vi "display_michelle_PKT_visjitter_stopadded_RandCont_PsuedoCO_TSLogFC2_ForTrainingLT.vi"() -> ()   [LabVIEW 2019]
uses:
  <vilib>/Analysis/Matrix/Datatypes/RealMatrix.ctl
  <vilib>/Utility/miscctls.llb/LVDateTimeRec.ctl
  <vilib>/Utility/file.llb/Write Delimited Spreadsheet (DBL).vi
  <vilib>/Analysis/Matrix/NI_Matrix.lvlib
panel:
  out "TimeStampTime":dbl
  out "initiatedlag":dbl
  out "date time rec":T1
  out "GlobalStartTime":i32
  out "JustStarted":i32
  out "LastTimeOutTime":dbl
  out "lambda":dbl
  out "maxITI":dbl
  out "minITI":dbl
  out "goEXP":dbl
  out "meanITI":dbl
  out "Lag1":dbl
  out "TSLog":dbl[][](array[numeric])
  out "TSLog2":dbl[][](array[numeric])
  out "Initialtime":dbl
  out "TSLog1":dbl[][](array[numeric])
  out "ArrayTemp3":T2
  out "StimID2":dbl
  out "Contrast":dbl
  out "TimeOutCounter":i32
  out "ElapsedTime_M":dbl
  out "Base_Contrast":dbl
  out "CurrentTrial":u32=1
  out "Jitter":dbl
  out "BaseITI":dbl
  out "VisStimDuration":dbl
  in  "Stop":bool
  out "Num trials":u32=204
  out "ISI Time":dbl
  out "Stim TS":dbl
  out "Output":dbl[][](array[numeric])
  out "Output frame":T2
  out "Array temp1":T2
  out "Elapsed Time":dbl
  out "Display":bool=TRUE
  out "Trial":u32=1
  out "reward":dbl[](array[numeric])
  out "stim_id":dbl[](array[numeric])
  out "stim_loaded":dbl
  out "Timings":dbl[](array[numeric])
  out "Stimuli Loaded?":bool
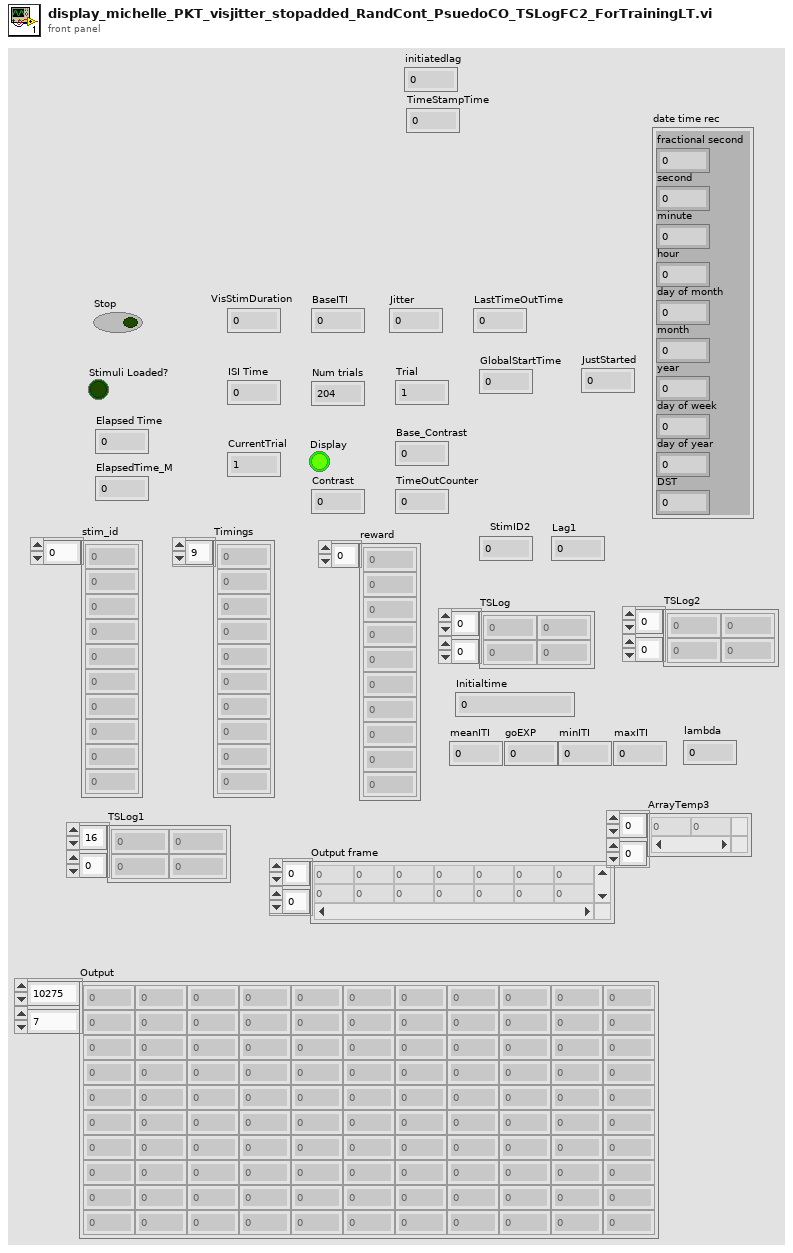
[diagram p1: front panel]
types:
  T1 = typedef "LVDateTimeRec.ctl" = cluster{"fractional second":dbl, "second":i32, "minute":i32, "hour":i32, "day of month":i32, "month":i32, "year":i32, "day of week":i32, "day of year":i32, "DST":i32}
  T2 = typedef "NI_Matrix.lvlib/RealMatrix.ctl" = dbl[][]
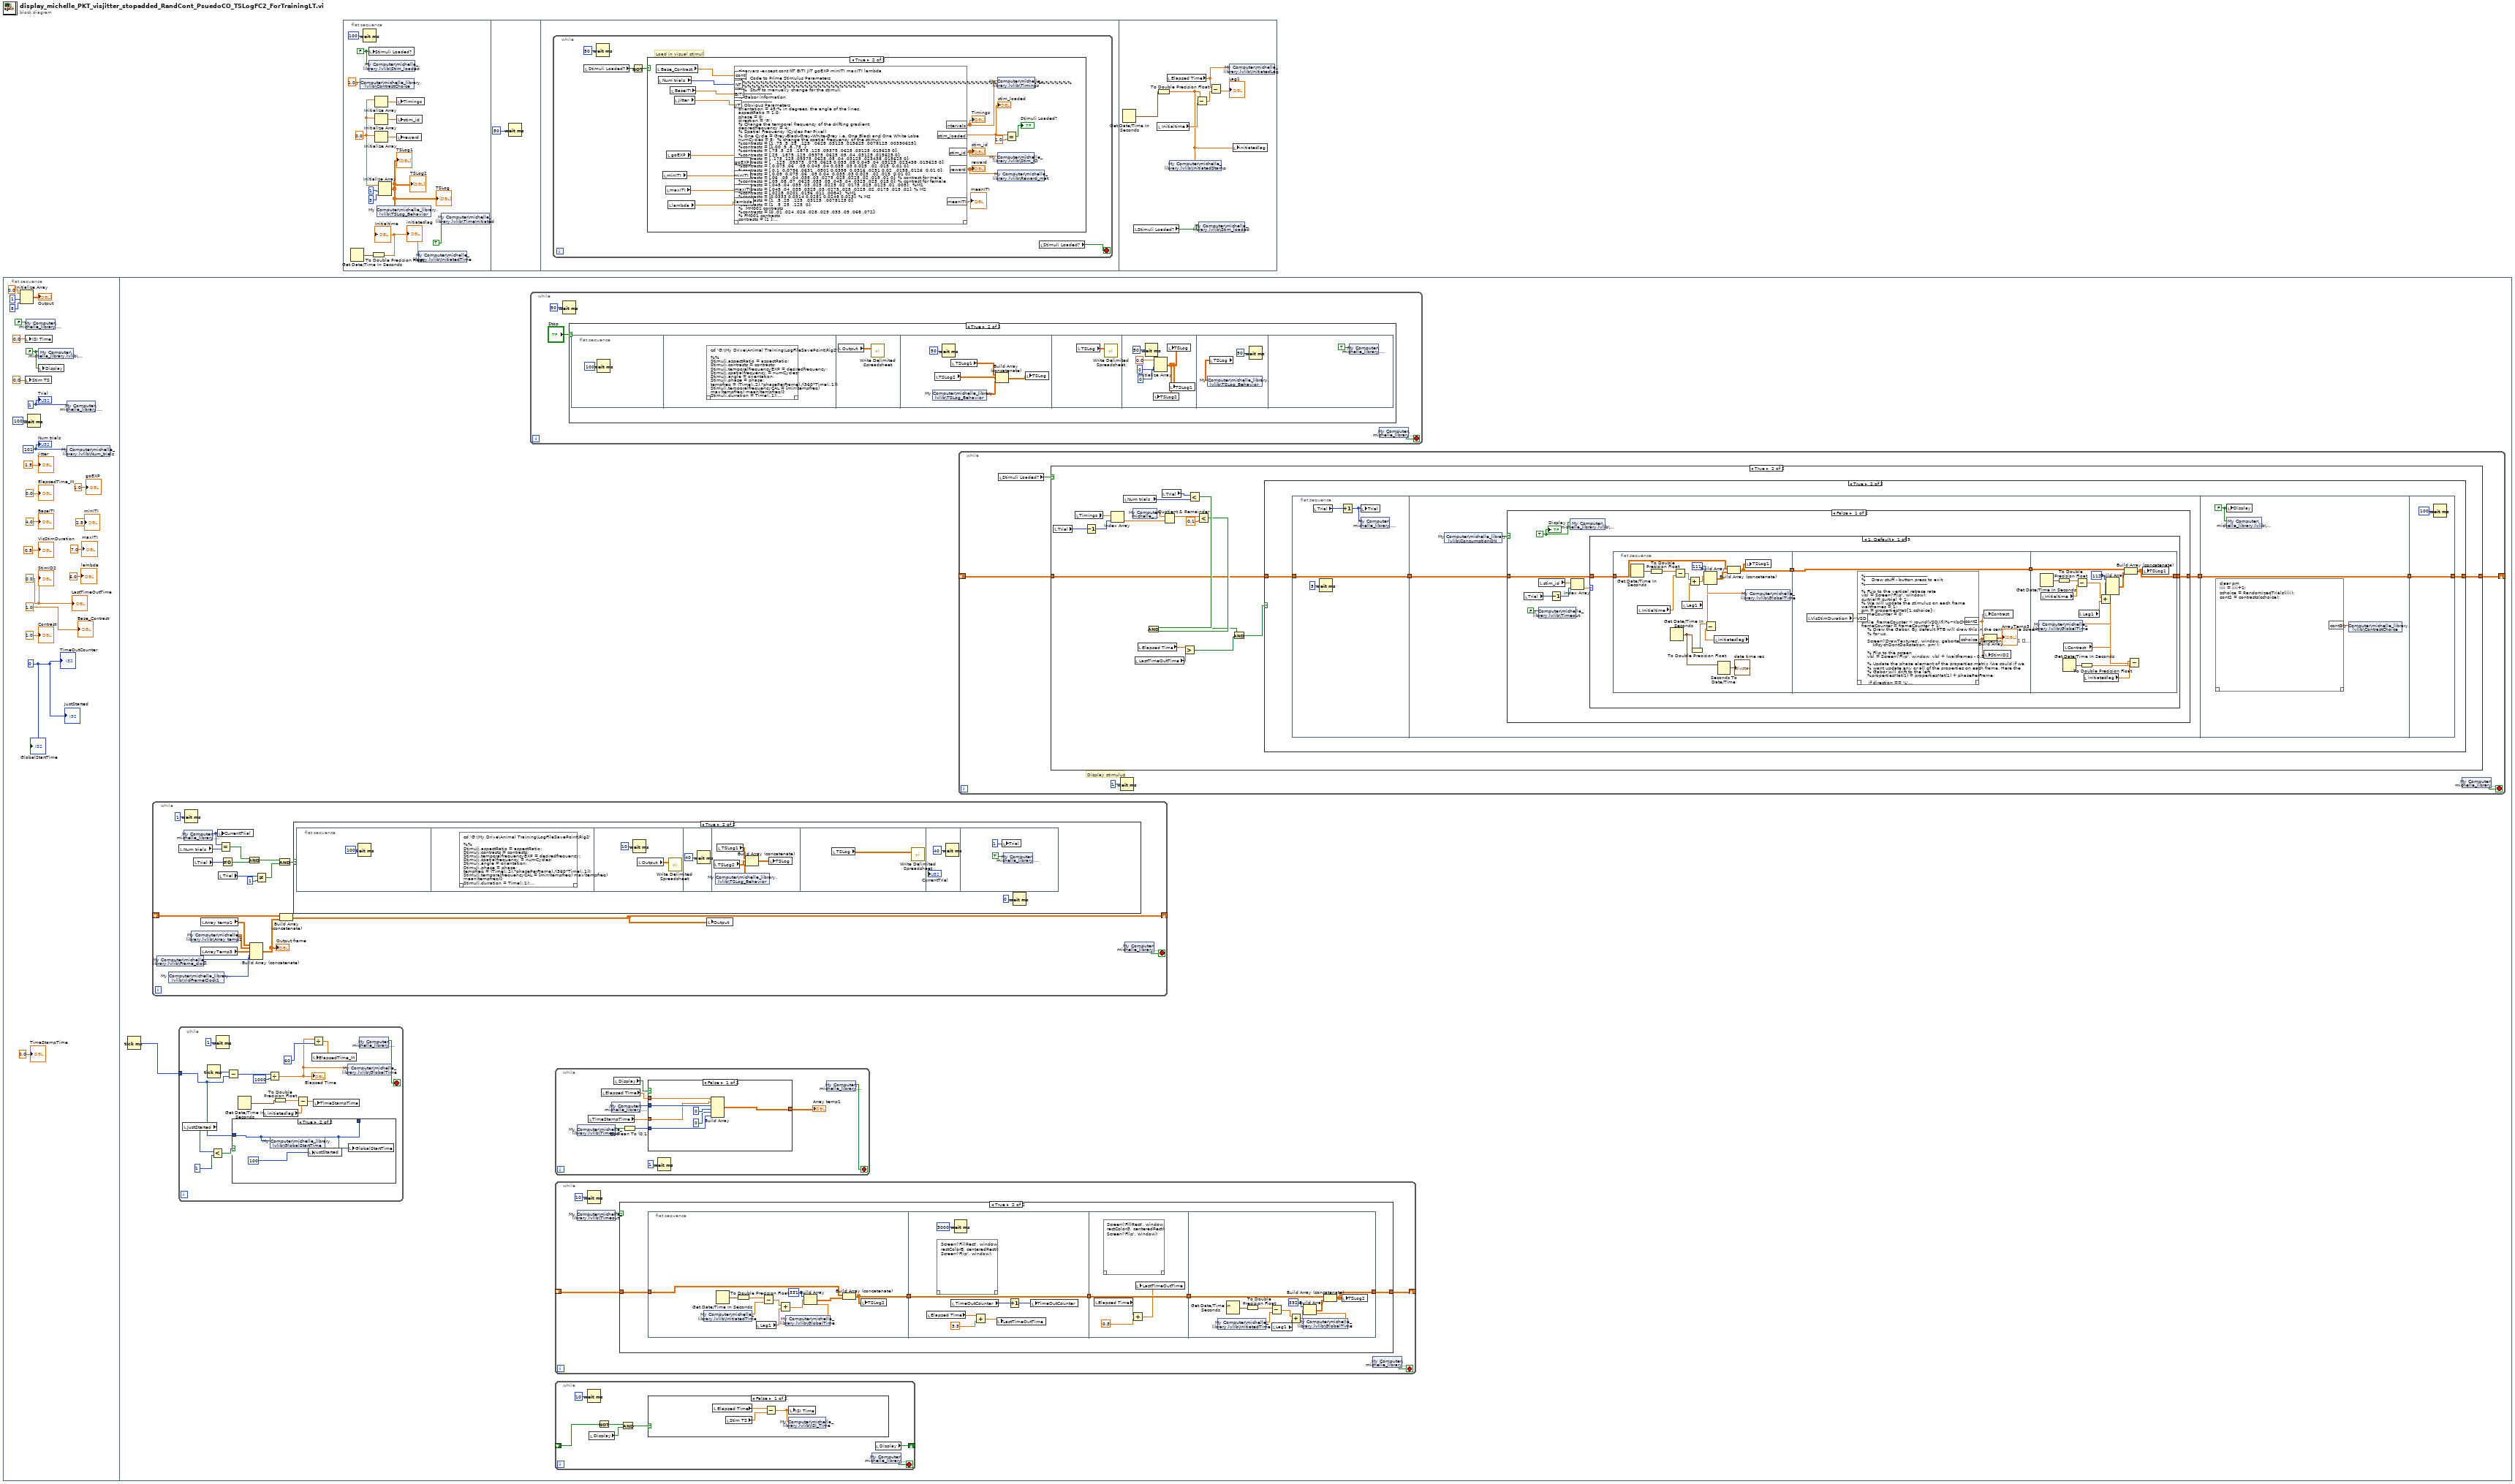
[diagram p0: block diagram]
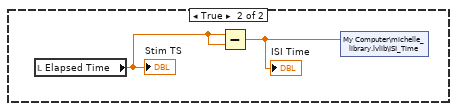
[diagram p5: hidden frame]
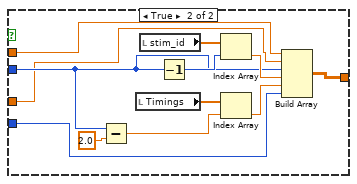
[diagram p6: hidden frame]
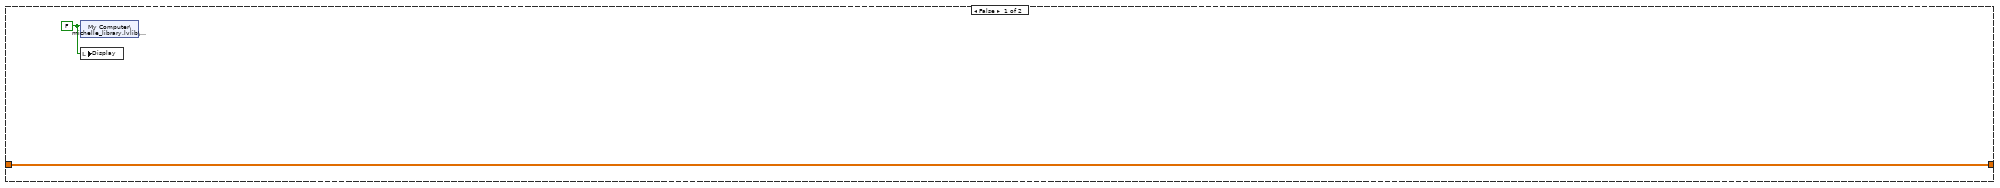
[diagram p10: hidden frame]
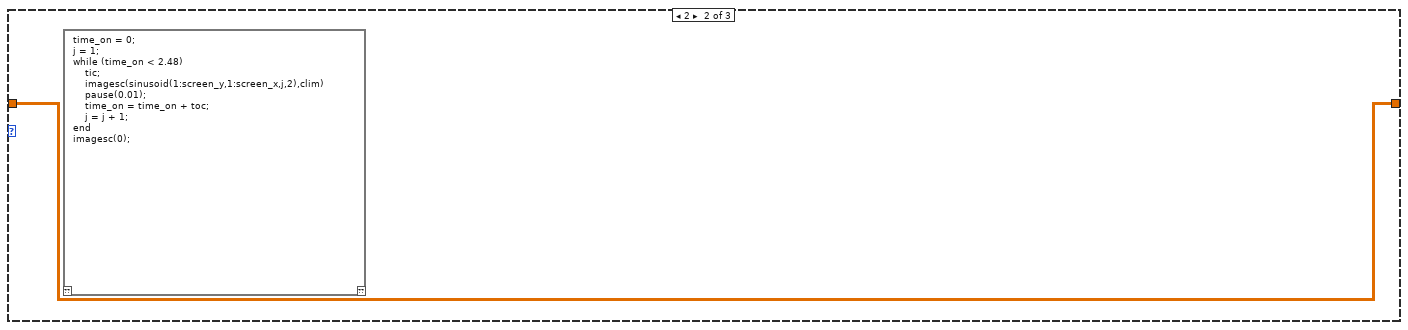
[diagram p11: hidden frame]
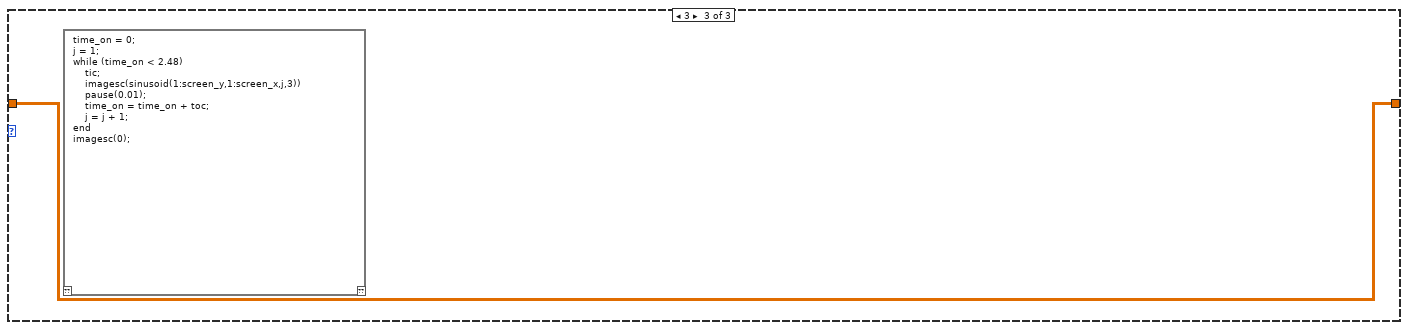
[diagram p12: hidden frame]
diagram:
  n1 = flat-sequence {
    frame #0 {
      w2 = 0.0
      w8 = 0
      w16 = u32 101
      w22 = FALSE ("Display")
      w24 = u32 1 ("Trial")
      n2 = Initialize Array(0.0 ("element"), 1 ("dimension size"), 8 ("dimension size")) -> (→"Output":dbl[][])
      n3 = local write "ISI Time"(0.0 ("ISI Time")) -> ()
      n4 = local write "Stim TS"(0.0 ("Stim TS")) -> ()
      n5 = shared-variable "My Computer\\michelle_library.lvlib\\Stop"(FALSE ("Stop")) -> ()  [unwired: 1 in, 1 out]
      n6 = Wait (ms)(milliseconds to wait=u32 100) -> ()  [unwired: 1 out]
      n7 = shared-variable "My Computer\\michelle_library.lvlib\\Display"(w22) -> ()  [unwired: 1 in, 1 out]
      n8 = local write "Display"(w22) -> ()
      n9 = shared-variable "My Computer\\michelle_library.lvlib\\Trial"(w24) -> ()  [unwired: 1 in, 1 out]
      n10 = shared-variable "My Computer\\michelle_library.lvlib\\Num_trials"(w16) -> ()  [unwired: 1 in, 1 out]
      "Trial" <- w24
      "Num trials" <- w16
      "VisStimDuration" <- 0.5
      "BaseITI" <- 4.0
      "Jitter" <- 1.5
      "Base_Contrast" <- 1.0
      "ElapsedTime_M" <- 0.0
      "TimeOutCounter" <- w8
      "Contrast" <- 1.0
      "StimID2" <- w2
      "goEXP" <- 1.0
      "minITI" <- 2.5
      "maxITI" <- 7.0
      "lambda" <- 6.0
      "LastTimeOutTime" <- w2
      "JustStarted" <- w8
      "GlobalStartTime" <- w8
      "TimeStampTime" <- 0.0
    }
    frame #1 {
      n11 = Tick Count (ms)() -> (millisecond timer value=w25:u32)
      n12 = while {
        shift-right: [w164] -> _
        shift-left: _ -> [w165]
        stop <- w167 stop-if-true
        n13 = shared-variable "My Computer\\michelle_library.lvlib\\Frame_clock"() -> (w149:u32)  [unwired: 1 in, 1 out]
        n14 = shared-variable "My Computer\\michelle_library.lvlib\\VidFrameClock1"() -> (w148:u32)  [unwired: 1 in, 1 out]
        n15 = local read "Num trials"() -> (w160:u32)
        n16 = shared-variable "My Computer\\michelle_library.lvlib\\Trial"() -> (w151:u32)  [unwired: 1 in, 1 out]
        n17 = Wait (ms)(milliseconds to wait=u32 1) -> ()  [unwired: 1 out]
        n18 = shared-variable "My Computer\\michelle_library.lvlib\\Array temp2"() -> (w162:dbl[][])  [unwired: 1 in, 1 out]
        n19 = local read "Trial"() -> (w158:u32)
        n20 = local read "Array temp1"() -> (w163:T2)
        n21 = local read "ArrayTemp3"() -> (w150:T2)
        n22 = local write "CurrentTrial"(w151) -> ()
        n23 = local read "Trial"() -> (w157:u32)
        n24 = Equal?(x=w151, y=w160) -> (x = y?=w159:bool)
        n25 = Not Equal To 0?(x=w158) -> (x != 0?=w154:bool)
        n26 = And(x=w159, y=w154) -> (x .and. y?=w152:bool)
        n27 = Build Array (concatenate)(w163, w162, w150, w149, w148) -> (w161:T2)
        "Output frame" <- w161
        n28 = Not Equal?(x=w157, y=1) -> (x != y?=w156:bool)
        n29 = And(x=w152, y=w156) -> (x .and. y?=w153:bool)
        n30 = Build Array (concatenate) ("Build Matrix")(w165, w161) -> (w164:T2)
        n31 = case shown="True" w153 {
          frame False {
          }
          frame True {
            n32 = flat-sequence {
              frame #0 {
                n33 = Wait (ms)(milliseconds to wait=100) -> ()  [unwired: 1 out]
              }
              frame #1 {
                n34 = script code="cd 'G:\\My Drive\\Animal Training\\LogFileSavePoint\\Rig2'\n\n%%\nStimuli.aspectRatio = aspectRatio;\nStimuli.contrasts = contrasts;\nStimuli.temporalfrequencyEXP = desiredfrequency;\nStimuli.spatialfrequency = numCycles;\nStimuli.angle = orientation;\nStimuli.phase = phase;\ntempfreq = (Time(:,2).*phasePerFrame)./(360*Time(:,1)); \nStimuli.temporalfrequencyCAL = [min(tempfreq) max(tempfreq) mean(tempfreq)];\nStimuli.durration = Time(:,1);\nStimuli.frames = Time(:,2);\nStimuli.contrast = Time(:,3);\nStimuli.intervals = intervals;\nif goEXP == 0\n     int.type = 'jitter';\n     int.baseITI = BITI;\n     int.jitter = JIT;\nelseif goEXP == 1\n     int.type = 'exponential';\n     int.minITI = minITI;\n     int.maxITI = maxITI;\n     int.lambda = lambda;\nend\nStimuli.IntervalData = int;\n\n\nWindow.Xpixels = screenXpixels;\nWindow.Ypixels = screenYpixels;\nWindow.Xcenter = xCenter;\nWindow.Ycenter = yCenter;\nWindow.ifi = ifi;\nWindow.screen = screenNumber;\n\n%%\n[logname] = generatelogname();\n\nsave(logname,'Stimuli','Window');"() -> ()  [unwired: 1 in, 1 out]
              }
              frame #2 {
                n35 = Wait (ms)(milliseconds to wait=u32 10) -> ()  [unwired: 1 out]
                n36 = local read "Output"() -> (w171:dbl[][])
                n37 = call-poly <vilib>:"Write Delimited Spreadsheet.vi"("2D data"=w171) -> ()  [unwired: 13 in, 2 out]
              }
              frame #3 {
                n38 = Wait (ms)(milliseconds to wait=u32 40) -> ()  [unwired: 1 out]
              }
              frame #4 {
                n39 = local read "TSLog2"() -> (w176:dbl[][])
                n40 = shared-variable "My Computer\\michelle_library.lvlib\\TSLog_Behavior"() -> (w174:dbl[][])  [unwired: 1 in, 1 out]
                n41 = local read "TSLog1"() -> (w175:dbl[][])
                n42 = Build Array (concatenate) ("Build Matrix")(w175, w176, w174) -> (w173:T2)
                n43 = local write "TSLog"(w173) -> ()
              }
              frame #5 {
                n44 = local read "TSLog"() -> (w177:dbl[][])
                n45 = call-poly <vilib>:"Write Delimited Spreadsheet.vi"("2D data"=w177) -> ()  [unwired: 13 in, 2 out]
              }
              frame #6 {
                n46 = Wait (ms)(milliseconds to wait=u32 40) -> ()  [unwired: 1 out]
              }
              frame #7 {
                n47 = local write "Trial"(1) -> ()
                n48 = shared-variable "My Computer\\michelle_library.lvlib\\Stop"(TRUE) -> ()  [unwired: 1 in, 1 out]
              }
            }
            n49 = Wait (ms)(milliseconds to wait=0) -> ()  [unwired: 1 out]
          }
        }
        n50 = local write "Output"(w164) -> ()
        n51 = shared-variable "My Computer\\michelle_library.lvlib\\Stop"() -> (w167:bool)  [unwired: 1 in, 1 out]
      }
      n52 = while {
        tunnel: w25 -> [w133]
        stop <- w140 stop-if-true
        n53 = local read "JustStarted"() -> (w135:i32)
        n54 = Tick Count (ms)() -> (millisecond timer value=w143:u32)
        n55 = Less?(x=w135, y=1) -> (x < y?=w136:bool)
        n56 = Wait (ms)(milliseconds to wait=u32 1) -> ()  [unwired: 1 out]
        n57 = Subtract(x=w143, y=w133) -> (x-y=w141:u32)
        n58 = case shown="True" w136 {
          tunnel: w133 -> [w145 w146]
          tunnel: [w145 w146] -> _
          frame False {
          }
          frame True {
            n59 = shared-variable "My Computer\\michelle_library.lvlib\\GlobalStartTime"(w146) -> ()  [unwired: 1 in, 1 out]
            n60 = local write "JustStarted"(100) -> ()
            n61 = local write "GlobalStartTime"(w146) -> ()
          }
        }
        n62 = Get Date/Time In Seconds() -> (seconds since 1Jan1904=w132:timestamp)
        n63 = local read "initiatedlag"() -> (w130:dbl)
        n64 = Divide(x=w141, y=u32 1000) -> (x/y=w137:dbl)
        "Elapsed Time" <- w137
        n65 = To Double Precision Float(number=w132) -> (double precision float=w129:dbl)
        n66 = Subtract(x=w129, y=w130) -> (x-y=w131:dbl)
        n67 = Divide(x=w137, y=60) -> (x/y=w138:dbl)
        n68 = local write "ElapsedTime_M"(w138) -> ()
        n69 = local write "TimeStampTime"(w131) -> ()
        n70 = shared-variable "My Computer\\michelle_library.lvlib\\GlobalTime"(w137) -> ()  [unwired: 1 in, 1 out]
        n71 = shared-variable "My Computer\\michelle_library.lvlib\\Stop"() -> (w140:bool)  [unwired: 1 in, 1 out]
      }
      n72 = while {
        stop <- w28 stop-if-true
        n73 = Wait (ms)(milliseconds to wait=50) -> ()  [unwired: 1 out]
        n74 = case shown="True" "Stop" {
          frame False {
          }
          frame True {
            n75 = flat-sequence {
              frame #0 {
                n76 = Wait (ms)(milliseconds to wait=100) -> ()  [unwired: 1 out]
              }
              frame #1 {
                n77 = script code="cd 'G:\\My Drive\\Animal Training\\LogFileSavePoint\\Rig2'\n\n%%\nStimuli.aspectRatio = aspectRatio;\nStimuli.contrasts = contrasts;\nStimuli.temporalfrequencyEXP = desiredfrequency;\nStimuli.spatialfrequency = numCycles;\nStimuli.angle = orientation;\nStimuli.phase = phase;\ntempfreq = (Time(:,2).*phasePerFrame)./(360*Time(:,1)); \nStimuli.temporalfrequencyCAL = [min(tempfreq) max(tempfreq) mean(tempfreq)];\nStimuli.durration = Time(:,1);\nStimuli.frames = Time(:,2);\nStimuli.contrast = Time(:,3);\nStimuli.intervals = intervals;\nif goEXP == 0\n     int.type = 'jitter';\n     int.baseITI = BITI;\n     int.jitter = JIT;\nelseif goEXP == 1\n     int.type = 'exponential';\n     int.minITI = minITI;\n     int.maxITI = maxITI;\n     int.lambda = lambda;\nend\nStimuli.IntervalData = int;\n\n\nWindow.Xpixels = screenXpixels;\nWindow.Ypixels = screenYpixels;\nWindow.Xcenter = xCenter;\nWindow.Ycenter = yCenter;\nWindow.ifi = ifi;\nWindow.screen = screenNumber;\n\n%%\n[logname] = generatelogname();\n\nsave(logname,'Stimuli','Window');"() -> ()  [unwired: 1 in, 1 out]
              }
              frame #2 {
                n78 = local read "Output"() -> (w30:dbl[][])
                n79 = call-poly <vilib>:"Write Delimited Spreadsheet.vi"("2D data"=w30) -> ()  [unwired: 13 in, 2 out]
              }
              frame #3 {
                n80 = shared-variable "My Computer\\michelle_library.lvlib\\TSLog_Behavior"() -> (w31:dbl[][])  [unwired: 1 in, 1 out]
                n81 = local read "TSLog2"() -> (w34:dbl[][])
                n82 = Wait (ms)(milliseconds to wait=50) -> ()  [unwired: 1 out]
                n83 = local read "TSLog1"() -> (w33:dbl[][])
                n84 = Build Array (concatenate) ("Build Matrix")(w33, w34, w31) -> (w32:T2)
                n85 = local write "TSLog"(w32) -> ()
              }
              frame #4 {
                n86 = local read "TSLog"() -> (w36:dbl[][])
                n87 = call-poly <vilib>:"Write Delimited Spreadsheet.vi"("2D data"=w36) -> ()  [unwired: 13 in, 2 out]
              }
              frame #5 {
                n88 = Wait (ms)(milliseconds to wait=50) -> ()  [unwired: 1 out]
                n89 = Initialize Array(0.0, 0, 0) -> (w38:dbl[][])
                n90 = local write "TSLog2"(w38) -> ()
                n91 = local write "TSLog"(w38) -> ()
                n92 = local write "TSLog1"(w38) -> ()
              }
              frame #6 {
                n93 = local read "TSLog"() -> (w43:dbl[][])
                n94 = shared-variable "My Computer\\michelle_library.lvlib\\TSLog_Behavior"(w43) -> ()  [unwired: 1 in, 1 out]
                n95 = Wait (ms)(milliseconds to wait=50) -> ()  [unwired: 1 out]
              }
              frame #7 {
                n96 = shared-variable "My Computer\\michelle_library.lvlib\\Stop"(TRUE) -> ()  [unwired: 1 in, 1 out]
              }
            }
          }
        }
        n97 = shared-variable "My Computer\\michelle_library.lvlib\\Stop"() -> (w28:bool)  [unwired: 1 in, 1 out]
      }
      n98 = while {
        stop <- w104 stop-if-true
        n99 = shared-variable "My Computer\\michelle_library.lvlib\\Timeout"() -> (w102:bool)  [unwired: 1 in, 1 out]
        n100 = local read "TimeStampTime"() -> (w101:dbl)
        n101 = local read "Elapsed Time"() -> (w108:dbl)
        n102 = shared-variable "My Computer\\michelle_library.lvlib\\Trial"() -> (w106:u32)  [unwired: 1 in, 1 out]
        n103 = local read "Display"() -> (w105:bool)
        n104 = Boolean To (0,1)(Boolean=w102) -> (0, 1=w103:i16)
        n105 = case shown="False" w105 {
          tunnel: w106 -> [w116 w120]
          tunnel: w108 -> [w110 w118]
          tunnel: [w115 w127] -> w107
          tunnel: w103 -> [w112 w122]
          tunnel: w101 -> [w111 w117]
          frame False {
            n106 = Build Array(w110, w111, w116, u32 0 ("milliseconds to wait"), 0, w112) -> (w115:T2)
          }
          frame True {
            n107 = Subtract(x=w120, y=2.0) -> (x-y=w119:dbl)
            n108 = local read "Timings"() -> (w125:dbl[])
            n109 = local read "stim_id"() -> (w128:dbl[])
            n110 = Decrement(x=w120) -> (x-1=w124:u32)
            n111 = Index Array(array=w128, index=w124) -> (element=w126:dbl)
            n112 = Index Array(array=w125, index=w119) -> (element=w123:dbl)
            n113 = Build Array(w118, w117, w120, w126, w123, w122) -> (w127:T2)
          }
        }
        "Array temp1" <- w107
        n114 = Wait (ms)(milliseconds to wait=u32 1) -> ()  [unwired: 1 out]
        n115 = shared-variable "My Computer\\michelle_library.lvlib\\Stop"() -> (w104:bool)  [unwired: 1 in, 1 out]
      }
      n116 = while {
        shift-right: [w45] -> _
        shift-left: _ -> [w46]
        stop <- w49 stop-if-true
        n117 = shared-variable "My Computer\\michelle_library.lvlib\\Timeout"() -> (w47:bool)  [unwired: 1 in, 1 out]
        n118 = Wait (ms)(milliseconds to wait=u32 10) -> ()  [unwired: 1 out]
        n119 = case shown="True" w47 {
          tunnel: w46 -> [w50 w55]
          tunnel: [w50 w54] -> w45
          frame False {
          }
          frame True {
            n120 = flat-sequence {
              tunnel: w55 -> [w61]
              tunnel: [w60] -> w52
              tunnel: [w70] -> w53
              tunnel: w52 -> [w70]
              tunnel: w53 -> [w77]
              tunnel: [w77] -> w51
              tunnel: [w82] -> w54
              tunnel: w51 -> [w83]
              frame #0 {
                n121 = shared-variable "My Computer\\michelle_library.lvlib\\InitiatedTime"() -> (w64:dbl)  [unwired: 1 in, 1 out]
                n122 = Get Date/Time In Seconds() -> (seconds since 1Jan1904=w66:timestamp)
                n123 = To Double Precision Float(number=w66) -> (double precision float=w65:dbl)
                n124 = local read "Lag1"() -> (w57:dbl)
                n125 = Subtract(x=w65, y=w64) -> (x-y=w58:dbl)
                n126 = Add(x=w58, y=w57) -> (x+y=w59:dbl)
                n127 = shared-variable "My Computer\\michelle_library.lvlib\\GlobalTime"() -> (w56:dbl)  [unwired: 1 in, 1 out]
                n128 = Build Array(331, w59, w56) -> (w63:T2)
                n129 = Build Array (concatenate) ("Build Matrix")(w61, w63) -> (w60:T2)
                n130 = local write "TSLog2"(w60) -> ()
              }
              frame #1 {
                n131 = local read "Elapsed Time"() -> (w67:dbl)
                n132 = script code="Screen('FillRect', window, rectColorB, centeredRect);\nScreen('Flip', window);"() -> ()  [unwired: 1 in, 1 out]
                n133 = local read "TimeOutCounter"() -> (w72:i32)
                n134 = Wait (ms)(milliseconds to wait=u32 3000) -> ()  [unwired: 1 out]
                n135 = Add(x=w67, y=3.3) -> (x+y=w69:dbl)
                n136 = local write "LastTimeOutTime"(w69) -> ()
                n137 = Increment(x=w72) -> (x+1=w71:i32)
                n138 = local write "TimeOutCounter"(w71) -> ()
              }
              frame #2 {
                n139 = local read "Elapsed Time"() -> (w76:dbl)
                n140 = script code="Screen('FillRect', window, rectColorG, centeredRect);\nScreen('Flip', window);"() -> ()  [unwired: 1 in, 1 out]
                n141 = Add(x=w76, y=0.3) -> (x+y=w75:dbl)
                n142 = local write "LastTimeOutTime"(w75) -> ()
              }
              frame #3 {
                n143 = shared-variable "My Computer\\michelle_library.lvlib\\InitiatedTime"() -> (w88:dbl)  [unwired: 1 in, 1 out]
                n144 = Get Date/Time In Seconds() -> (seconds since 1Jan1904=w86:timestamp)
                n145 = To Double Precision Float(number=w86) -> (double precision float=w87:dbl)
                n146 = Subtract(x=w87, y=w88) -> (x-y=w80:dbl)
                n147 = local read "Lag1"() -> (w79:dbl)
                n148 = Add(x=w80, y=w79) -> (x+y=w81:dbl)
                n149 = shared-variable "My Computer\\michelle_library.lvlib\\GlobalTime"() -> (w78:dbl)  [unwired: 1 in, 1 out]
                n150 = Build Array(332, w81, w78) -> (w84:T2)
                n151 = Build Array (concatenate) ("Build Matrix")(w83, w84) -> (w82:T2)
                n152 = local write "TSLog2"(w82) -> ()
              }
            }
          }
        }
        n153 = shared-variable "My Computer\\michelle_library.lvlib\\Stop"() -> (w49:bool)  [unwired: 1 in, 1 out]
      }
      n154 = while {
        shift-right: [w93] -> _
        shift-left: _ -> [w92]
        stop <- w95 stop-if-true
        n155 = Wait (ms)(milliseconds to wait=u32 10) -> ()  [unwired: 1 out]
        n156 = local read "Display"() -> (w90:bool)
        n157 = Not(x=w92) -> (.not. x?=w91:bool)
        n158 = And(x=w91, y=w90) -> (x .and. y?=w89:bool)
        n159 = case shown="False" w89 {
          frame False {
            n160 = local read "Elapsed Time"() -> (w96:dbl)
            n161 = local read "Stim TS"() -> (w98:dbl)
            n162 = Subtract(x=w96, y=w98) -> (x-y=w97:dbl)
            n163 = local write "ISI Time"(w97) -> ()
            n164 = shared-variable "My Computer\\michelle_library.lvlib\\ISI_Time"(w97) -> ()  [unwired: 1 in, 1 out]
          }
          frame True {
            n165 = local read "Elapsed Time"() -> (w99:dbl)
            "Stim TS" <- w99
            n166 = Subtract(x=w99, y=w99) -> (x-y=w100:dbl)
            "ISI Time" <- w100
            n167 = shared-variable "My Computer\\michelle_library.lvlib\\ISI_Time"(w100) -> ()  [unwired: 1 in, 1 out]
          }
        }
        n168 = shared-variable "My Computer\\michelle_library.lvlib\\Stop"() -> (w95:bool)  [unwired: 1 in, 1 out]
        n169 = local read "Display"() -> (w93:bool)
      }
      n170 = while {
        shift-right: [w181] -> _
        shift-left: _ -> [w182]
        stop <- w184 stop-if-true
        # "Display stimulus"
        n171 = local read "Stimuli Loaded?"() -> (w183:bool)
        n172 = case shown="True" w183 {
          tunnel: w182 -> [w186 w193]
          tunnel: [w186 w192] -> w181
          frame False {
          }
          frame True {
            n173 = local read "Trial"() -> (w194:u32)
            n174 = local read "Timings"() -> (w202:dbl[])
            n175 = Decrement(x=w194) -> (x-1=w195:u32)
            n176 = Index Array(array=w202, index=w195) -> (element=w201:dbl)
            n177 = local read "Num trials"() -> (w197:u32)
            n178 = shared-variable "My Computer\\michelle_library.lvlib\\ISI"() -> (w196:dbl)  [unwired: 1 in, 1 out]
            n179 = local read "LastTimeOutTime"() -> (w188:dbl)
            n180 = local read "Elapsed Time"() -> (w187:dbl)
            n181 = local read "Trial"() -> (w200:u32)
            n182 = Quotient & Remainder(x=w196, y=w201) -> (x-y*floor(x/y)=w204:dbl)  [unwired: 1 out]
            n183 = Greater?(x=w187, y=w188) -> (0:w189:bool)
            n184 = Less?(x=w200, y=w197) -> (x < y?=w199:bool)
            n185 = Less?(x=w204, y=0.1) -> (x < y?=w198:bool)
            n186 = And(x=w199, y=w198) -> (x .and. y?=w191:bool)
            n187 = And(x=w191, y=w189) -> (x .and. y?=w190:bool)
            n188 = case shown="True" w190 {
              tunnel: w193 -> [w205 w210]
              tunnel: [w205 w209] -> w192
              frame False {
                w206 = FALSE ("Display")
                n189 = shared-variable "My Computer\\michelle_library.lvlib\\Display"(w206) -> ()  [unwired: 1 in, 1 out]
                n190 = local write "Display"(w206) -> ()
              }
              frame True {
                n191 = flat-sequence {
                  tunnel: [w212] -> w211
                  tunnel: w210 -> [w212]
                  tunnel: w211 -> [w217]
                  tunnel: [w216] -> w207
                  tunnel: [w271] -> w208
                  tunnel: w207 -> [w271]
                  tunnel: [w274] -> w209
                  tunnel: w208 -> [w274]
                  frame #0 {
                    n192 = local read "Trial"() -> (w215:u32)
                    n193 = Wait (ms)(milliseconds to wait=u32 5) -> ()  [unwired: 1 out]
                    n194 = Increment(x=w215) -> (x+1=w214:u32)
                    n195 = local write "Trial"(w214) -> ()
                    n196 = shared-variable "My Computer\\michelle_library.lvlib\\Trial"(w214) -> ()  [unwired: 1 in, 1 out]
                  }
                  frame #1 {
                    n197 = shared-variable "My Computer\\michelle_library.lvlib\\ConsumptionON"() -> (w218:bool)  [unwired: 1 in, 1 out]
                    n198 = case shown="False" w218 {
                      tunnel: w217 -> [w220 w270]
                      tunnel: [w219 w270] -> w216
                      frame False {
                        w221 = TRUE ("Boolean")
                        n199 = local read "Trial"() -> (w224:u32)
                        n200 = shared-variable "My Computer\\michelle_library.lvlib\\Timeout"(FALSE) -> ()  [unwired: 1 in, 1 out]
                        n201 = local read "stim_id"() -> (w226:dbl[])
                        n202 = Decrement(x=w224) -> (x-1=w223:u32)
                        n203 = shared-variable "My Computer\\michelle_library.lvlib\\Display"(w221) -> ()  [unwired: 1 in, 1 out]
                        n204 = Index Array(array=w226, index=w223) -> (element=w225:dbl)
                        n205 = case shown="1, Default" w225 {
                          tunnel: w220 -> [w230 w268 w269]
                          tunnel: [w229 w268 w269] -> w219
                          frame 1, Default {
                            n206 = flat-sequence {
                              tunnel: w230 -> [w245]
                              tunnel: [w244] -> w228
                              tunnel: w228 -> [w247]
                              tunnel: [w247] -> w227
                              tunnel: [w266] -> w229
                              tunnel: w227 -> [w265]
                              frame #0 {
                                n207 = Get Date/Time In Seconds() -> (seconds since 1Jan1904=w242:timestamp)
                                n208 = local read "Initialtime"() -> (w240:dbl)
                                n209 = To Double Precision Float(number=w242) -> (double precision float=w241:dbl)
                                n210 = Get Date/Time In Seconds() -> (seconds since 1Jan1904=w235:timestamp)
                                n211 = Subtract(x=w241, y=w240) -> (x-y=w238:dbl)
                                n212 = local read "Lag1"() -> (w239:dbl)
                                n213 = Add(x=w238, y=w239) -> (x+y=w237:dbl)
                                n214 = To Double Precision Float(number=w235) -> (double precision float=w233:dbl)
                                n215 = local read "initiatedlag"() -> (w231:dbl)
                                n216 = Subtract(x=w233, y=w231) -> (x-y=w232:dbl)
                                n217 = Seconds To Date/Time(time stamp (now)=w235) -> (date time rec=→"date time rec":T1)  [unwired: 1 in]
                                n218 = shared-variable "My Computer\\michelle_library.lvlib\\GlobalTime"() -> (w236:dbl)  [unwired: 1 in, 1 out]
                                n219 = Build Array(111, w237, w236, w232) -> (w243:T2)
                                n220 = Build Array (concatenate) ("Build Matrix")(w245, w243) -> (w244:T2)
                                n221 = local write "TSLog1"(w244) -> ()
                              }
                              frame #1 {
                                n222 = local read "VisStimDuration"() -> (w249:dbl)
                                n223 = script code="%------------------------------------------\n%    Draw stuff - button press to exit\n%------------------------------------------\n\n% FLip to the vertical retrace rate\nvbl = Screen('Flip', window);\ncurtrial= curtrial + 1;\n% We will update the stimulus on each frame\nwaitframes = 1;\npm = propertiesMat{1,cchoice};\nframeCounter = 0;\ntic\nwhile  frameCounter < round(VSD/ifi)%~KbCheck\nframeCounter = frameCounter + 1;\n    % Draw the Gabor. By default PTB will draw this in the center of the screen\n    % for us.\n   \n    Screen('DrawTextures', window, gabortex, [], [], orientation, [], [], [], [],...\n        kPsychDontDoRotation, pm');\n\n    % Flip to the screen\n    vbl = Screen('Flip', window, vbl + (waitframes - 0.5) * ifi);\n\n    % Update the phase element of the properties matrix (we could if we\n    % want update any or all of the properties on each frame. Here the\n    % Gabor will drift to the left.\n    %propertiesMat(1) = propertiesMat(1) + phasePerFrame;\n \n     if direction == 'L'\n          pm(1) = pm(1) + phasePerFrame;\n     elseif direction =='R'\n          pm(1) = pm(1) - phasePerFrame;\n     end\n\nend\nTime(curtrial,1) = toc;\nTime(curtrial,2) = frameCounter;\nTime(curtrial,3) = pm(4);\nvbl = Screen('Flip', window);"("VSD"=w249) -> ("cont2"=w251:dbl, "cchoice"=w250:dbl)  [unwired: 1 in, 1 out]
                                n224 = local write "Contrast"(w251) -> ()
                                n225 = Build Array(w251, w250) -> (→"ArrayTemp3":T2)
                                n226 = local write "StimID2"(w250) -> ()
                              }
                              frame #2 {
                                n227 = shared-variable "My Computer\\michelle_library.lvlib\\GlobalTime"() -> (w257:dbl)  [unwired: 1 in, 1 out]
                                n228 = Get Date/Time In Seconds() -> (seconds since 1Jan1904=w263:timestamp)
                                n229 = local read "Initialtime"() -> (w262:dbl)
                                n230 = To Double Precision Float(number=w263) -> (double precision float=w261:dbl)
                                n231 = Get Date/Time In Seconds() -> (seconds since 1Jan1904=w255:timestamp)
                                n232 = local read "Contrast"() -> (w256:dbl)
                                n233 = Subtract(x=w261, y=w262) -> (x-y=w260:dbl)
                                n234 = local read "Lag1"() -> (w258:dbl)
                                n235 = To Double Precision Float(number=w255) -> (double precision float=w254:dbl)
                                n236 = local read "initiatedlag"() -> (w252:dbl)
                                n237 = Add(x=w260, y=w258) -> (x+y=w259:dbl)
                                n238 = Subtract(x=w254, y=w252) -> (x-y=w253:dbl)
                                n239 = Build Array(112, w259, w257, w256, w253) -> (w267:T2)
                                n240 = Build Array (concatenate) ("Build Matrix")(w265, w267) -> (w266:T2)
                                n241 = local write "TSLog1"(w266) -> ()
                              }
                            }
                          }
                          frame 2 {
                            n242 = script code="time_on = 0;\nj = 1;\nwhile (time_on < 2.48)\n    tic;\n    imagesc(sinusoid(1:screen_y,1:screen_x,j,2),clim)\n    pause(0.01);\n    time_on = time_on + toc;\n    j = j + 1;\nend\nimagesc(0);"() -> ()  [unwired: 1 in, 1 out]
                          }
                          frame 3 {
                            n243 = script code="time_on = 0;\nj = 1;\nwhile (time_on < 2.48)\n    tic;\n    imagesc(sinusoid(1:screen_y,1:screen_x,j,3))\n    pause(0.01);\n    time_on = time_on + toc;\n    j = j + 1;\nend\nimagesc(0);"() -> ()  [unwired: 1 in, 1 out]
                          }
                        }
                        "Display" <- w221
                      }
                      frame True {
                      }
                    }
                  }
                  frame #2 {
                    w273 = FALSE ("Display")
                    n244 = script code="clear pm\niiii = iiii+1;\ncchoice = RandomizedTrials(iiii);\ncont2 = contrasts(cchoice);"() -> ("cont2"=w272:dbl)  [unwired: 1 in, 1 out]
                    n245 = local write "Display"(w273) -> ()
                    n246 = shared-variable "My Computer\\michelle_library.lvlib\\Display"(w273) -> ()  [unwired: 1 in, 1 out]
                    n247 = shared-variable "My Computer\\michelle_library.lvlib\\ContrastChoice"(w272) -> ()  [unwired: 1 in, 1 out]
                  }
                  frame #3 {
                    n248 = Wait (ms)(milliseconds to wait=u32 100) -> ()  [unwired: 1 out]
                  }
                }
              }
            }
          }
        }
        n249 = Wait (ms)(milliseconds to wait=u32 1) -> ()  [unwired: 1 out]
        n250 = shared-variable "My Computer\\michelle_library.lvlib\\Stop"() -> (w184:bool)  [unwired: 1 in, 1 out]
      }
    }
  }
  n251 = flat-sequence {
    frame #0 {
      w282 = 0.0 ("element")
      w284 = FALSE ("Stimuli Loaded?")
      n252 = Get Date/Time In Seconds() -> (seconds since 1Jan1904=w279:timestamp)
      n253 = shared-variable "My Computer\\michelle_library.lvlib\\ContrastChoice"(1.0) -> ()  [unwired: 1 in, 1 out]
      n254 = Wait (ms)(milliseconds to wait=u32 100) -> ()  [unwired: 1 out]
      n255 = local write "Stimuli Loaded?"(w284) -> ()
      n256 = shared-variable "My Computer\\michelle_library.lvlib\\Stim_loaded"(w284) -> ()  [unwired: 1 in, 1 out]
      n257 = To Double Precision Float(number=w279) -> (double precision float=w278:dbl)
      "Initialtime" <- w278
      "initiatedlag" <- w278
      n258 = Initialize Array(w282) -> (w287:dbl[])  [unwired: 1 in]
      n259 = Initialize Array(w282) -> (w286:dbl[])  [unwired: 1 in]
      n260 = Initialize Array(w282) -> (w285:dbl[])  [unwired: 1 in]
      n261 = Initialize Array(w282, 1, 3) -> (w276:dbl[][])
      "TSLog1" <- w276
      "TSLog2" <- w276
      "TSLog" <- w276
      n262 = shared-variable "My Computer\\michelle_library.lvlib\\TSLog_Behavior"(w276) -> ()  [unwired: 1 in, 1 out]
      n263 = local write "Timings"(w287) -> ()
      n264 = local write "stim_id"(w286) -> ()
      n265 = local write "reward"(w285) -> ()
      n266 = shared-variable "My Computer\\michelle_library.lvlib\\InitiatedTime"(w278) -> ()  [unwired: 1 in, 1 out]
      n267 = shared-variable "My Computer\\michelle_library.lvlib\\TimeInitiated"(TRUE) -> ()  [unwired: 1 in, 1 out]
    }
    frame #1 {
      n268 = Wait (ms)(milliseconds to wait=u32 50) -> ()  [unwired: 1 out]
    }
    frame #2 {
      n269 = while {
        stop <- w290 stop-if-true
        # "Load in visual stimuli"
        n270 = local read "Stimuli Loaded?"() -> (w292:bool)
        n271 = Wait (ms)(milliseconds to wait=u32 50) -> ()  [unwired: 1 out]
        n272 = Not(x=w292) -> (.not. x?=w291:bool)
        n273 = case shown="True" w291 {
          frame False {
          }
          frame True {
            n274 = local read "Base_Contrast"() -> (w300:dbl)
            n275 = local read "Num trials"() -> (w303:u32)
            n276 = local read "minITI"() -> (w296:dbl)
            n277 = local read "maxITI"() -> (w295:dbl)
            n278 = local read "goEXP"() -> (w297:dbl)
            n279 = local read "lambda"() -> (w294:dbl)
            n280 = local read "BaseITI"() -> (w302:dbl)
            n281 = local read "Jitter"() -> (w301:dbl)
            n282 = script code="clearvars -except cont NT BITI JIT goEXP minITI maxITI lambda\n\n%%  Code to Prime Stimulus Parameters\n%%%%%%%%%%%%%%%%%%%%%%%%%%%%%%%%%%%%%%%%%%%%%%%%%%%%%%%%%%%%%%%%%%%%%%%%%%%%%%%%%%%%%%%%%%%%%%%%%%%%%%%%%\n%%  Stuff to manually change for the stimuli\n%--------------------\n% Gabor information\n%--------------------\n% Obvious Parameters\norientation = 45;% in degrees, the angle of the lines.\naspectRatio = 1.0;\nphase = 0;\ndirection = 'R';\n% Change the temporal frequency of the drifting gradient\ndesiredfrequency = 4;\n% Spatial Frequency (Cycles Per Pixel)\n% One Cycle = Grey-Black-Grey-White-Grey i.e. One Black and One White Lobe\nnumCycles = 8;  % change the spatial frequency of the stimuli\n%contrasts = [1 .75 .5 .25  .125  .0625 .03125 .015625 .0078125 .00390625];\n%contrasts = [1.00 .9 .8 .75  ];\n%contrasts = [.75 .5 .25  .1875 .125 .09375 .0625 .03125 .015625 0];\n%contrasts = [.25  .1875 .125 .09375 .0625 .05 .04 .03125 .015625 0];\n%contrasts = [ .175 .125 .09375 .0625 .05 .04 .03125 .023438 .015625 0];\n%contrasts = [   .125  .09375  .075 .0625 0.055 .05 0.045 .04 .03125 .023438 .015625 0];\n%contrasts = [ 0.075 .06   .05 0.045 .04 0.035 .03 0.025  .02 .015  0.01 0];\n%contrasts = [ 0.1  0.0796 .0631  .0501 0.0398  0.0316 .0251 0.02  .0158 .0126  0.01 0];\n%contrasts = [ 0.09  0.075 .06  .05 0.04  0.035 .03 0.025  .02 .015  0.01 0];\n%contrasts = [.06  .05  .04 .035 .03 .0275 .025 .0225 .02 .015 .01 0]; % contrast for male\n%contrasts = [.09 .08 .07 .0625 .055 .05 .045 .04 .0325 .025 .015 0]; % contrast for female\n%contrasts = [.045 .04 .035 .03 .025 .0225 .02 .0175 .015 .0125 .01 .005];  %M1\n%contrasts = [.045 .04 .035 .0325 .03 .0275 .025 .0225 .02 .0175 .015 .01]; % M2\n%contrasts = [.0228 .0201 .0156 .011 .0084];  %M1\n%contrasts = [0.0333 0.0314 0.0281 0.0248 0.023]; % M2\n%contrasts = [1  .5 .25  .125  .03125  .0078125 0];\n%contrasts = [1  .5 .25  .125  0];\n%  MM001 contrasts\n%contrasts = [0 .01 .024 .026 .028 .029 .033 .05 .068 .072];\n% FM001 contrasts\ncontrasts = [1 ];\n\ngo = 1;\nmaxc = round(numel(contrasts)/2);\n%%  To be run of not using exponential\n%%%%%%%%%%%%%%%%%%%%%%%%%%%%%%%%%%%%%%%%%%%%%%%%%%%%%%%%%%%%%%%%%%%%%%%%%%%%%%%%%%%%%%\n% This code will randomize the order of contrasts being presented\n[RandomizedTrials]=RandomizeTrials_Psuedo_function(contrasts,NT,'n');\n\n% This code will generate inter trial intervals with either random jitter\n% or based on an exponential distribution\nif goEXP < 1\n     jit = JIT;\n     jitter = rand(1,NT);\n     jitter = 2*jit*(jitter- .5);\n     ITIbase = BITI;\n     intervals = [ones(1,NT)*ITIbase];\n     intervals = intervals + jitter;\nelseif goEXP > 0\n     intervals = exponentialITI(1/lambda, minITI, maxITI, NT);\nend\n\n%%  Prep the stimulus presentation software\n%%%%%%%%%%%%%%%%%%%%%%%%%%%%%%%%%%%%%%%%%%%%%%%%%%%%%%%%%%%%%%%%%%%%%%%%%%%\nScreen('Preference', 'SkipSyncTests', 1);\nsca;\nclose all;\n% Setup PTB with some default values\nPsychDefaultSetup(2);\n% Set the screen number to the external secondary monitor if there is one connected\nscreenNumber = max(Screen('Screens'));\n\n% Define black, white and grey\nwhite = WhiteIndex(screenNumber);\nblack = BlackIndex(screenNumber);\ngrey = white / 2;\n\n% Open the screen & define it's dimensions\n[window, windowRect] = PsychImaging('OpenWindow', screenNumber, grey,...\n    [], 32, 2, [], [], kPsychNeedRetinaResolution);\n[screenXpixels, screenYpixels] = Screen('WindowSize', window);\n[xCenter, yCenter] = RectCenter(windowRect);\n\n% Get the vertical refresh rate of the monitor\nifi = Screen('GetFlipInterval', window);\n\n% Set maximum priority level\ntopPriorityLevel = MaxPriority(window);\nPriority(topPriorityLevel);\n\n\n% Build a procedural gabor texture (Note: to get a \"standard\" Gabor patch\n% we set a grey background offset, disable normalisation, and set a\n% pre-contrast multiplier of 0.5).\n% Dimension of the region where will draw the Gabor in pixels\ngaborDimPix = windowRect(3);\n% Sigma of Gaussian  (how much to fade around the edges)\nsigma = gaborDimPix / 0;  % change the 0 value to alter the fading\nphasePerFrame = desiredfrequency*360*ifi;\nfreq = numCycles / gaborDimPix;\n\nbackgroundOffset = [0.5 0.5 0.5 0.0];\ndisableNorm = 1;\npreContrastMultiplier = 0.5;\ngabortex = CreateProceduralGabor(window, gaborDimPix, gaborDimPix, [],...\n    backgroundOffset, disableNorm, preContrastMultiplier);\n\n% Randomise the phase of the Gabors and make a properties matrix.\nfor N = 1:numel(contrasts)\npropertiesMat{1,N} = [phase, freq, sigma, contrasts(N), aspectRatio, 0, 0, 0];\nend\n\niiii = 1;\ncchoice = RandomizedTrials(iiii);\ncont2 = contrasts(cchoice);\npm = propertiesMat{1,1};\ncurtrial = 0;\n\n%%  Build up the rectangles for the pause and hold screen\nbaseRect = [0 0 screenXpixels screenYpixels];\ncenteredRect = CenterRectOnPointd(baseRect, xCenter, yCenter);\nrectColorB = [0 0 0];\nrectColorG = [128 128 128]/255;\n\n%%  Finalize the trial data and orders\nstim_id = [ones(1,NT)*1];\nreward = [ones(1,NT)*1];\nmeanITI = nanmean(intervals);\nrand_idx1 = randperm(NT);\nrand_idx2 = randperm(NT);\nintervals = intervals(rand_idx2);\nstim_id = stim_id(rand_idx2);\nreward = reward(rand_idx2);\n%%  All Done!\n%  indicate that the necessary preloading of data has been completed.\nstim_loaded = 1;" ("Script Node")("NT"=w303, "BITI"=w302, "JIT"=w301, "cont"=w300, "goEXP"=w297, "minITI"=w296, "maxITI"=w295, "lambda"=w294) -> ("stim_loaded"=w308:dbl, "intervals"=w304:dbl[], "stim_id"=w305:dbl[], "reward"=w306:dbl[], "meanITI"=→"meanITI":dbl)  [unwired: 1 in, 1 out]
            "stim_loaded" <- w308
            "Timings" <- w304
            "stim_id" <- w305
            "reward" <- w306
            n283 = shared-variable "My Computer\\michelle_library.lvlib\\Timings"(w304) -> ()  [unwired: 1 in, 1 out]
            n284 = shared-variable "My Computer\\michelle_library.lvlib\\Stim_ID"(w305) -> ()  [unwired: 1 in, 1 out]
            n285 = shared-variable "My Computer\\michelle_library.lvlib\\Reward_mat"(w306) -> ()  [unwired: 1 in, 1 out]
            n286 = Equal?(x=w308, y=1.0) -> (x = y?=→"Stimuli Loaded?":bool)
          }
        }
        n287 = local read "Stimuli Loaded?"() -> (w290:bool)
      }
    }
    frame #3 {
      n288 = Get Date/Time In Seconds() -> (seconds since 1Jan1904=w315:timestamp)
      n289 = local read "Stimuli Loaded?"() -> (w311:bool)
      n290 = To Double Precision Float(number=w315) -> (double precision float=w309:dbl)
      n291 = local read "Initialtime"() -> (w314:dbl)
      n292 = local read "Elapsed Time"() -> (w310:dbl)
      n293 = shared-variable "My Computer\\michelle_library.lvlib\\InitiatedStamp"(w309) -> ()  [unwired: 1 in, 1 out]
      n294 = Subtract(x=w309, y=w314) -> (x-y=w313:dbl)
      n295 = shared-variable "My Computer\\michelle_library.lvlib\\Stim_loaded"(w311) -> ()  [unwired: 1 in, 1 out]
      n296 = Subtract(x=w310, y=w313) -> (x-y=→"Lag1":dbl)
      n297 = shared-variable "My Computer\\michelle_library.lvlib\\InitiatedLag"(w310) -> ()  [unwired: 1 in, 1 out]
      n298 = local write "initiatedlag"(w309) -> ()
    }
  }
